vi "Host.Test.vi"() -> ()   [LabVIEW 2020]
uses:
  <vilib>/rvi/interface/nirviOpenFPGA/nirviOpenFPGA.xnode
  <vilib>/rvi/interface/nirviMethod/nirviMethod.xnode
  <vilib>/rvi/interface/nirviCloseFPGA/nirviCloseFPGA.xnode
  <vilib>/rvi/errors/niLvFpgaMergeErrorWithErrorCode.vi
  <vilib>/FPGAPlugInAG/Dynamic/niLvFpga_ReadFifo_Dynamic.vi
  <vilib>/FPGAPlugInAG/Dynamic/niLvFpga_WriteFifo_Dynamic.vi
  <vilib>/FPGAPlugInAG/Dynamic/niLvFpga_Close_Dynamic.vi
  <instrlib>/_niInstr/Network/Types/v1/MAC Address.ctl
  <instrlib>/_niInstr/Network/Types/v1/niInstr Network Types v1.lvlib
  <instrlib>/_niInstr/Network/Types/v1/IPv4 Address.ctl
  <vilib>/rvi/interface/nirviReadWriteControl/nirviReadWriteControl.xnode
  NiFpgaLv.dll
  <vilib>/Utility/error.llb/Error Cluster From Error Code.vi
  <vilib>/rvi/interface/Simulation/niFpgaSimulationCallBeginRW.vi
  <vilib>/rvi/errors/niLvFpgaAdjustHostInterfaceError.vi
  arty/test/fpga.test.harness.vi
panel:
  in  "Use PCap":bool
  in  "String":string="00, 0a, 35, 00, 01, 02, 60, a4, 4c, 63, f7, ea, 08, 00, 45, 00, 00, 5a, cb, 2a, 00, 00, 80, 11, eb, 11, c0, a8, 01, ca, c0, a8, 01, 3c, fb, 46, 17, 71, 00, 46, 19, 41, 54, 68, 69, 73, 20, 69, 73, 20, 74, 68, 65, 20, 6d, 65, 73, 73, 61, 67, 65, 2e, 20, 49, 74, 20, 77, 69, 6c, 6c, 20, 62, 65, 20, 72, 65, 70, 65, 61, 74, 65, 64, 2e, 20, 20, 54, 6f, 20, 47, 65, 6e, 65, 73, 79, 73, 20, 6f, 72, 20, 41, 72, 74, 79, 2e, 25, 7e, 94, 9c, "
  out "data string":string
  out "Data":u8[](array[numeric]) format="%.0x"
  out "error out":errorcluster
  in  "error in":errorcluster
  out "Array":u16[](array[numeric])
  in  "PCap File":string="data.pcap"
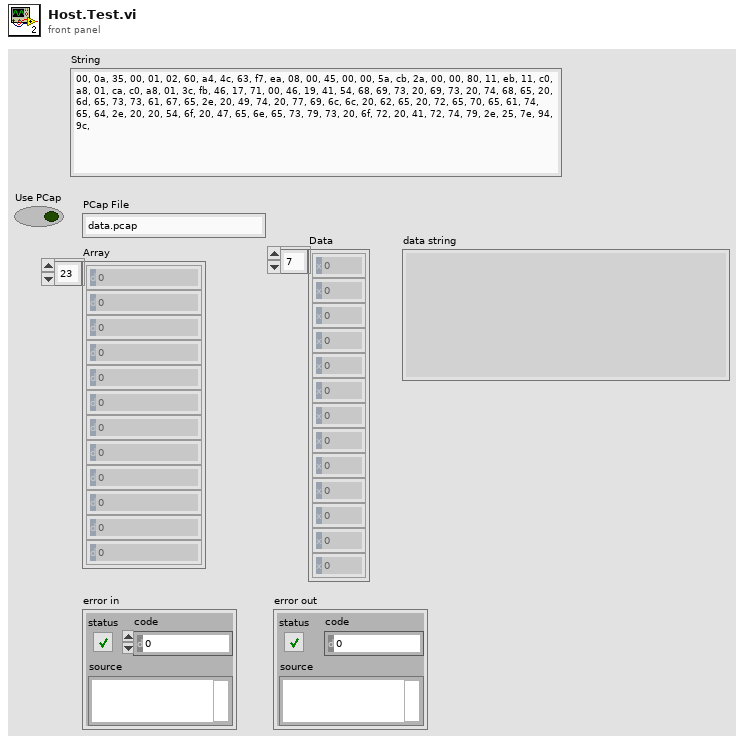
[diagram p1: front panel]
types:
  T1 = typedef "niInstr Network Types v1.lvlib/IPv4 Address.ctl" = u8[]
  T2 = typedef "niInstr Network Types v1.lvlib/MAC Address.ctl" = u8[]
  T3 = typedef "record.ctl" = cluster{"ts_sec":u32, "ts_usec":u32, "incl_len":u32, "orig_len":u32, "payload":u8[]}
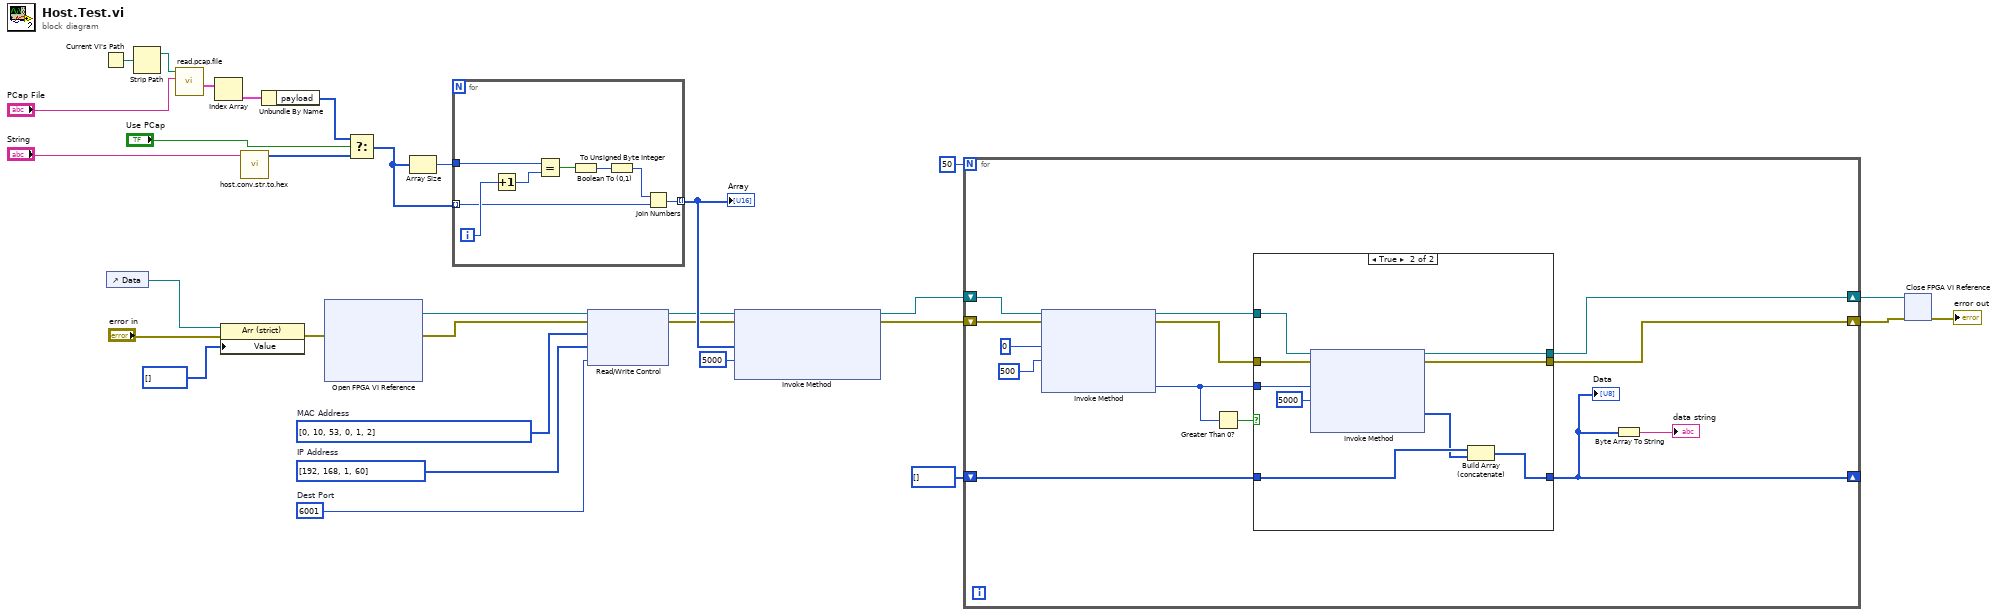
[diagram p0: block diagram]
diagram:
  w7 = u16 6001  # Dest Port
  w6 = T1 [192, 168, 1, 60]  # IP Address
  w8 = T2 [0, 10, 53, 0, 1, 2]  # MAC Address
  n1 = Current VI's Path() -> (path=w31:path)
  n2 = control-ref of="Data"() -> (w15:refnum<vi>)
  n3 = Strip Path(path=w31) -> (stripped path=w30:path)  [unwired: 1 out]
  n4 = call "read.pcap.file.vi"("PCap File"="PCap File", "Path"=w30) -> ("Records"=w28:T3[])  [unwired: 7 in, 2 out]
  n5 = Index Array(array=w28) -> (element=w27:T3)  [unwired: 1 in]
  n6 = property class="Arr (strict)"(reference=w15, error in="error in", "Value"=u8[] []) -> (error out=w12:errorcluster)  [unwired: 1 out]
  n7 = call "host.conv.str.to.hex.vi"("String"="String") -> ("Array 2"=w2:u8[])  [unwired: 10 in]
  n8 = Unbundle By Name(w27) -> ("payload"=w4:u8[])
  n9 = xnode "Open FPGA VI Reference"("error in"=w12) -> ("FPGA VI Reference Out"=w25:refnum<k20>, "error out"=w10:errorcluster)  [unwired: 1 in]
  n10 = Select(t=w4, s="Use PCap", f=w2) -> (s? t:f=w3:u8[])
  n11 = Array Size(array=w3) -> (size(s)=w26:i32)
  n12 = for {
    tunnel: w3 -> [w37] mode=indexing
    tunnel: w26 -> [w39]
    tunnel: [w33] -> w24 mode=indexing
    i -> [w38]
    n13 = Increment(x=w38) -> (x+1=w32:i32)
    n14 = Equal?(x=w39, y=w32) -> (x = y?=w36:bool)
    n15 = Boolean To (0,1)(Boolean=w36) -> (0, 1=w35:i16)
    n16 = To Unsigned Byte Integer(number=w35) -> (unsigned 8bit integer=w34:u8)
    n17 = Join Numbers(hi=w34, lo=w37) -> ((hi.lo)=w33:u16)
  }
  "Array" <- w24
  n18 = xnode "Read/Write Control"("FPGA VI Reference In"=w25, "error in"=w10, "MAC Address"=w8, "IP Address"=w6, "Dest Port"=w7) -> ("FPGA VI Reference Out"=w11:refnum<k20>, "error out"=w9:errorcluster)
  n19 = xnode "Invoke Method"("FPGA VI Reference In"=w11, "error in"=w9, "Data"=w24, "Timeout (ms)"=5000) -> ("FPGA VI Reference Out"=w21:refnum<k20>, "error out"=w20:errorcluster)  [unwired: 1 out]
  n20 = for {
    N: 50 -> [_]
    shift-right: [w41] -> _
    shift-left: u8[] [] ("Data") -> [w45]
    shift-right: [w44] -> w17
    shift-left: w21 -> [w52]
    shift-right: [w43] -> w16
    shift-left: w20 -> [w51]
    n21 = xnode "Invoke Method"("FPGA VI Reference In"=w52, "error in"=w51, "Number of Elements"=u32 0, "Timeout (ms)"=500) -> ("FPGA VI Reference Out"=w46:refnum<k20>, "error out"=w42:errorcluster, "Elements Remaining"=w47:u32)  [unwired: 1 out]
    n22 = Greater Than 0?(x=w47) -> (x > 0?=w48:bool)
    n23 = case shown="True" w48 {
      tunnel: w47 -> [_ w64]
      tunnel: w46 -> [w54 w62]
      tunnel: [w55 w59] -> w41
      tunnel: w45 -> [w55 w61]
      tunnel: [w54 w58] -> w44
      tunnel: [w53 w57] -> w43
      tunnel: w42 -> [w53 w56]
      frame False {
      }
      frame True {
        n24 = xnode "Invoke Method"("FPGA VI Reference In"=w62, "error in"=w56, "Number of Elements"=w64, "Timeout (ms)"=5000) -> ("FPGA VI Reference Out"=w58:refnum<k20>, "error out"=w57:errorcluster, "Data"=w60:u8[])  [unwired: 1 out]
        n25 = Build Array (concatenate)(w61, w60) -> (w59:u8[])
      }
    }
    "Data" <- w41
    n26 = Byte Array To String(unsigned byte array=w41) -> (string=→"data string":string)
  }
  n27 = xnode "Close FPGA VI Reference"("FPGA VI Reference In"=w17, "error in"=w16) -> ("error out"=→"error out":errorcluster)
